vi "EIT_Demod.vi"(6 "Reshape size":i32=-1, 7 "Search Width %":dbl=0.1, 10 "Frequencies":dbl[](array[numeric]), 11 "Waveforms":waveform(dbl)[](array[waveform])) -> (1 "FreqsOut":dbl[][](array[numeric]), 2 "Amp2D":dbl[][](array[numeric]), 3 "Amp1D":dbl[](array[numeric]))   [LabVIEW 2020]
uses:
  <vilib>/measure/matone.llb/Extract Single Tone Information N Chan.vi
  <vilib>/measure/NI_MAPro.lvlib
panel:
  out "Reshape size Out":i32
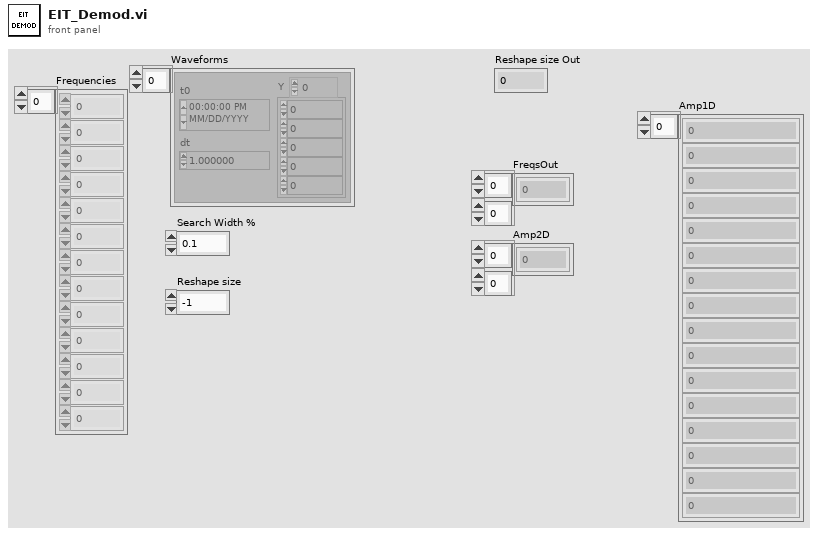
[diagram p1: front panel]
types:
  T1 = cluster{"approx freq. (optional)":dbl, "Search Width %":dbl}
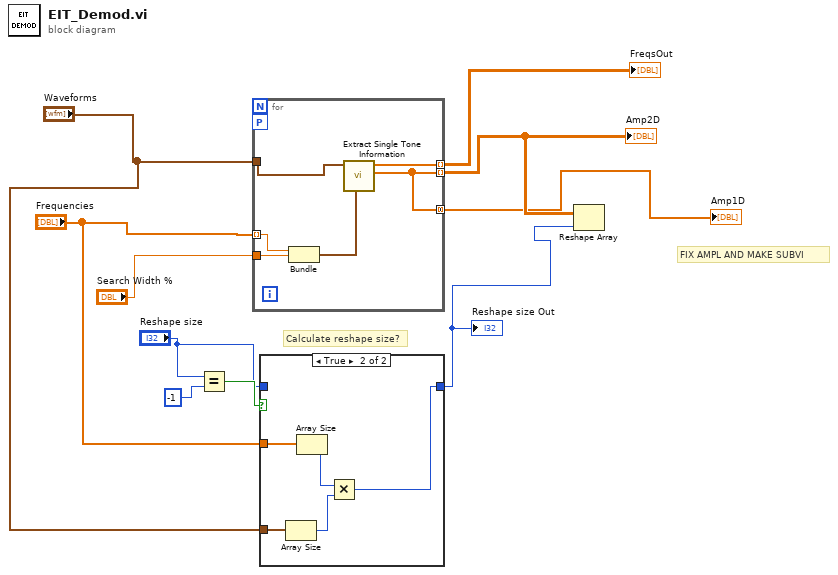
[diagram p0: block diagram]
diagram:
  # "FIX AMPL AND MAKE SUBVI"
  # "Calculate reshape size?"
  n1 = Equal?(x="Reshape size", y=-1) -> (x = y?=w6:bool)
  n2 = for {
    tunnel: "Waveforms" -> [w16]
    tunnel: [w15] -> w10 mode=indexing
    tunnel: [w11] -> w9 mode=indexing
    tunnel: "Frequencies" -> [w13] mode=indexing
    workers-P: _ -> [_]
    tunnel: "Search Width %" -> [w12]
    tunnel: [w11] -> w1 mode=concatenating
    n3 = Bundle("approx freq. (optional)"=w13, "Search Width %"=w12) -> (w14:T1)  [unwired: 1 in]
    n4 = call-poly <vilib>:"Extract Single Tone Information.vi"("advanced search"=w14, "time signals in"=w16) -> ("detected amplitudes"=w11:dbl[], "detected frequencies"=w15:dbl[])  [unwired: 4 in, 4 out]
  }
  "FreqsOut" <- w10
  "Amp2D" <- w9
  "Amp1D" <- w1
  n5 = case shown="True" w6 {
    tunnel: "Reshape size" -> [w17 _]
    tunnel: [w17 w18] -> w4
    tunnel: "Frequencies" -> [_ w21]
    tunnel: "Waveforms" -> [_ w20]
    frame False {
    }
    frame True {
      n6 = Array Size(array=w20) -> (size(s)=w19:i32)
      n7 = Array Size(array=w21) -> (size(s)=w22:i32)
      n8 = Multiply(x=w22, y=w19) -> (x*y=w18:i32)
    }
  }
  "Reshape size Out" <- w4
  n9 = Reshape Array(w9, w4) -> ()  [unwired: 1 out]
